vi "Get FIFO Flags.vi"(11 "Debug Flags in":refnum<class "Debug Flags.lvclass">) -> (2 "FIFO":refnum<class "FIFO Flags.lvclass">, 3 "Debug Flags out":refnum<class "Debug Flags.lvclass">)   [LabVIEW 2017, in "DSF Core.lvlib" / "Debug Flags.lvclass"]
uses:
  Debug Flags.lvclass
  FIFO Flags/FIFO Flags.lvclass
  Debug Flags.lvclass/Debug Flags.ctl
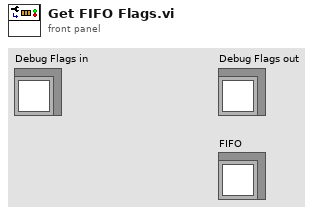
[diagram p1: front panel]
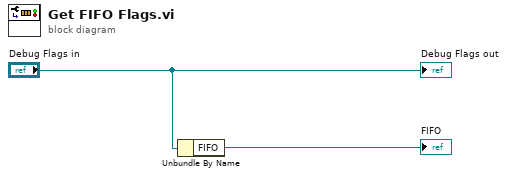
[diagram p0: block diagram]
diagram:
  n1 = Unbundle By Name("Debug Flags in") -> ("FIFO"=→"FIFO":refnum<class "FIFO Flags.lvclass">)
  "Debug Flags out" <- "Debug Flags in"
